vi "CAN Messw. Pegasor,Semtech.vi"() -> (2 "CAN data":T1[](array[typedef])=[{"timestamp"=timestamp(0 s since 1904-01-01), "payload"=[0, 2, 3, 4, 5, 6, 7, 8], "identifier"=2, "type"=0, "extended?"=FALSE, "echo?"=FALSE}, {"timestamp"=timestamp(0 s since 1904-01-01), "payload"=[0, 1, 2, 3, 4, 5, 6, 7], "identifier"=3, "type"=0, "extended?"=FALSE, "echo?"=FALSE}] {"payload" format="%x"; "timestamp" format="%<%.7X\n%x>T"; "type" items=["CAN Data"=0, "CAN Remote"=1, "CAN Bus Error"=2, "CAN 2.0 Data"=8, "CAN FD Data"=16, "CAN FD+BRS Data"=24, "J1939 Data"=192, "Delay"=224, "Log Trigger"=225, "Start Trigger"=226]; "identifier" format="%x"})   [LabVIEW 2020]
uses:
  195161_2023-03-15/cRIO/CAN Interface/CAN Interface.lvlib
  FGV CAN Daten Aktionen.ctl
  Messdaten/Aktionen FGV Messwerte zusammenfassen.ctl
  195161_2023-03-15/Messdaten/Messdaten.lvlib
  <vilib>/xnet/xnet.llb/XNET Frame Type CAN.ctl
  <vilib>/xnet/xnet.llb/XNET Frame CAN.ctl
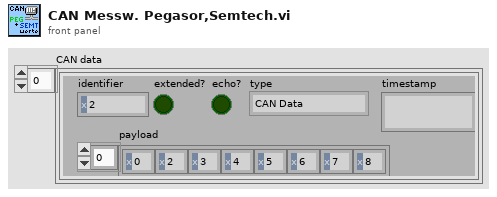
[diagram p1: front panel]
types:
  T1 = typedef "XNET Frame CAN.ctl" = cluster{"timestamp":timestamp, "payload":u8[], "identifier":u32, "type":T2, "extended?":bool, "echo?":bool}
  T2 = typedef "XNET Frame Type CAN.ctl" = u8
  T3 = typedef "Messdaten.lvlib/Aktionen FGV Messwerte zusammenfassen.ctl" = enum16{"lesen", "FT-IR", "Algebraic", "LabBaseName", "LabBaseNr"}
  T4 = typedef "CAN Interface.lvlib/FGV CAN Daten Aktionen.ctl" = enum16{"lesen", "Daten", "Konfig", "laden", "speichern", "Status"}
  T5 = typedef "Statusübersicht.lvlib/Aktion Status Analysatoren.ctl" = enum16{"lesen", "initialisieren", "Analysatoren aktiv", "FAS 1 Fehler", "FAS 2 Fehler", "FAS 3 Fehler", "MS 1 Fehler", "MS 2 Fehler", "MS 3 Fehler", "Mi3 1 Fehler", "Mi3 2 Fehler", "Mi3 3 Fehler", "DS Fehler", "Felder einfärben"}
  T6 = typedef "Statusübersicht.lvlib/Status.ctl" = cluster{"FAS 1 aktiv":bool, "FAS 1 Fehler":bool, "FAS 2 aktiv":bool, "FAS 2 Fehler":bool, "FAS 3 aktiv":bool, "FAS 3 Fehler":bool, "MS 1 aktiv":bool, "MS 1 Fehler":bool, "MS 2 aktiv":bool, "MS 2 Fehler":bool, "MS 3 aktiv":bool, "MS 3 Fehler":bool, "Mi3 1 aktiv":bool, "Mi3 1 Fehler":bool, "Mi3 2 aktiv":bool, "Mi3 2 Fehler":bool, "Mi3 3 aktiv":bool, "Mi3 3 Fehler":bool, "DS aktiv":bool, "DS Fehler":bool}
  T7 = typedef "CAN Konfig.lvlib/Konfig Daten PC.ctl" = cluster{"Baude Rate":T8, "COM state":u8, "Frame-ID FTIR Start":u32, "Frame-ID FTIR End":u32, "Frame-ID Status Start":u32, "Frame-ID Status End":u32, "Zustand Information":u32, "Aktion":u32, "Frame-ID FTIR Arry":u32[], "Frame-ID Status Arry":u32[], "GPS Start":u32, "Interface":refnum<k21>}
  T8 = typedef "CAN Interface.lvlib/Baude Rate.ctl" = u32
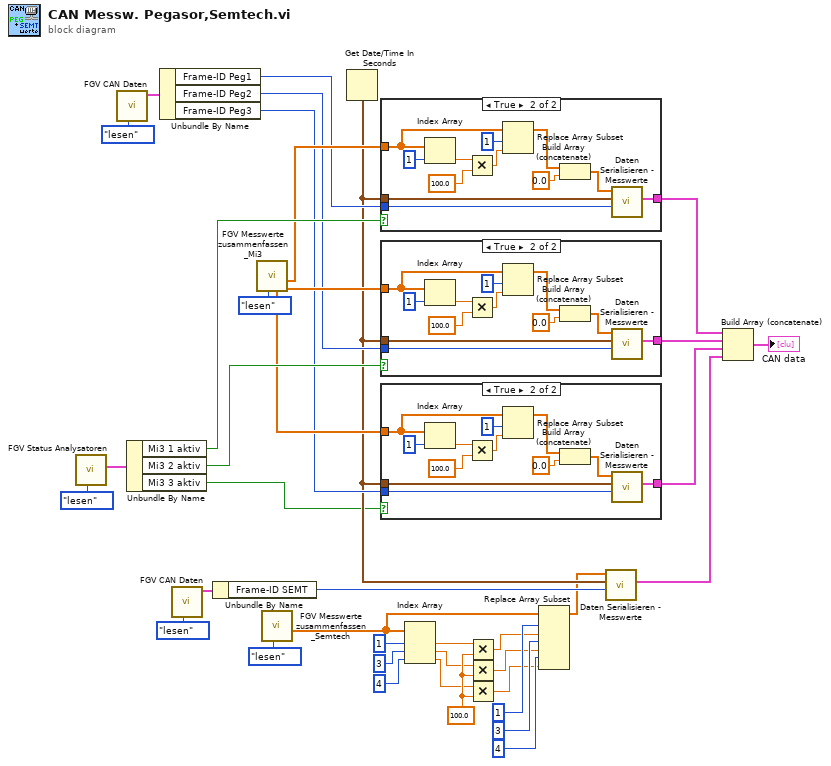
[diagram p0: block diagram]
diagram:
  w8 = sgl 100.0
  n1 = call "FGV Status Analysatoren.vi"("Aktionen"=Aktion_Status_Analysatoren."lesen") -> ("Status Analysatoren"=w35:T6)  [unwired: 10 in]
  n2 = call "FGV CAN Daten.vi"("Aktionen"=FGV_CAN_Daten_Aktionen."lesen") -> ("Konfig Daten"=w38:T7)  [unwired: 8 in, 2 out]
  n3 = Unbundle By Name(w35) -> ("Mi3 1 aktiv"=w34:bool, "Mi3 2 aktiv"=w23:bool, "Mi3 3 aktiv"=w19:bool)
  n4 = Unbundle By Name(w38) -> ("Frame-ID Peg1"=w32:u32, "Frame-ID Peg2"=w24:u32, "Frame-ID Peg3"=w21:u32)
  n5 = call "FGV CAN Daten.vi"("Aktionen"=FGV_CAN_Daten_Aktionen."lesen") -> ("Konfig Daten"=w27:T7)  [unwired: 8 in, 2 out]
  n6 = Unbundle By Name(w27) -> ("Frame-ID SEMT"=w29:u32)
  n7 = call "FGV Messwerte zusammenfassen_Mi3.vi"("Aktionen"=Aktionen_FGV_Messwerte_zusammenfassen."lesen") -> ("Messwerte Mi3 2"=w25:sgl[], "Messwerte Mi3 1"=w33:sgl[], "Messwerte Mi3 3"=w22:sgl[])  [unwired: 5 in, 3 out]
  n8 = call "FGV Messwerte zusammenfassen_Semtech.vi"("Aktionen"=Aktionen_FGV_Messwerte_zusammenfassen."lesen") -> ("Messwerte"=w13:sgl[])  [unwired: 9 in, 1 out]
  n9 = Get Date/Time In Seconds() -> (seconds since 1Jan1904=w20:timestamp)
  n10 = case shown="True" w34 {
    tunnel: [_ w51] -> w31
    tunnel: w33 -> [_ w41]
    tunnel: w20 -> [_ w50]
    tunnel: w32 -> [_ w49]
    frame False {
    }
    frame True {
      n11 = Index Array(array=w41, index=1 ("Index")) -> (element=w44:sgl)
      n12 = Multiply(x=w44, y=sgl 100.0) -> (x*y=w46:sgl)
      n13 = Replace Array Subset(array=w41, new element=w46, index=1 ("Index")) -> (w40:sgl[])
      n14 = Build Array (concatenate)(w40, sgl 0.0) -> (w47:sgl[])
      n15 = call "Daten Serialisieren - Messwerte.vi"("Frame-ID"=w49, "Aktuelle Zeit"=w50, "Messdaten"=w47) -> ("data"=w51:T1[])  [unwired: 8 in]
    }
  }
  n16 = case shown="True" w23 {
    tunnel: [_ w63] -> w17
    tunnel: w25 -> [_ w53]
    tunnel: w20 -> [_ w62]
    tunnel: w24 -> [_ w61]
    frame False {
    }
    frame True {
      n17 = Index Array(array=w53, index=1 ("Index")) -> (element=w56:sgl)
      n18 = Multiply(x=w56, y=sgl 100.0) -> (x*y=w58:sgl)
      n19 = Replace Array Subset(array=w53, new element=w58, index=1 ("Index")) -> (w52:sgl[])
      n20 = Build Array (concatenate)(w52, sgl 0.0) -> (w59:sgl[])
      n21 = call "Daten Serialisieren - Messwerte.vi"("Frame-ID"=w61, "Aktuelle Zeit"=w62, "Messdaten"=w59) -> ("data"=w63:T1[])  [unwired: 8 in]
    }
  }
  n22 = case shown="True" w19 {
    tunnel: [_ w75] -> w18
    tunnel: w22 -> [_ w65]
    tunnel: w20 -> [_ w74]
    tunnel: w21 -> [_ w73]
    frame False {
    }
    frame True {
      n23 = Index Array(array=w65, index=1 ("Index")) -> (element=w68:sgl)
      n24 = Multiply(x=w68, y=sgl 100.0) -> (x*y=w70:sgl)
      n25 = Replace Array Subset(array=w65, new element=w70, index=1 ("Index")) -> (w64:sgl[])
      n26 = Build Array (concatenate)(w64, sgl 0.0) -> (w71:sgl[])
      n27 = call "Daten Serialisieren - Messwerte.vi"("Frame-ID"=w73, "Aktuelle Zeit"=w74, "Messdaten"=w71) -> ("data"=w75:T1[])  [unwired: 8 in]
    }
  }
  n28 = Index Array(array=w13, index #1=1 ("Index"), index #2=3 ("Index"), index #3=4 ("Index")) -> (element #1=w14:sgl, element #2=w7:sgl, element #3=w6:sgl)
  n29 = Multiply(x=w14, y=w8) -> (x*y=w3:sgl)
  n30 = Multiply(x=w7, y=w8) -> (x*y=w2:sgl)
  n31 = Multiply(x=w6, y=w8) -> (x*y=w4:sgl)
  n32 = Replace Array Subset(array=w13, new element #1=w3, index #1=1 ("Index"), new element #2=w2, index #2=3 ("Index"), new element #3=w4, index #3=4 ("Index")) -> (w1:sgl[])
  n33 = call "Daten Serialisieren - Messwerte.vi"("Frame-ID"=w29, "Aktuelle Zeit"=w20, "Messdaten"=w1) -> ("data"=w26:T1[])  [unwired: 8 in]
  n34 = Build Array (concatenate)(w31, w17, w18, w26) -> (→"CAN data":T1[])
